vi "SELECCION_MODO_INGENIERIA.vi"(7 "EST_3":bool, 8 "EST_2":bool, 9 "EST_1":bool) -> (3 "MOV eSTADO":i32)   [LabVIEW 2019, in "Class 2.lvclass"]
uses:
  Class 2.lvclass
panel:
  out "ESTADO":i8
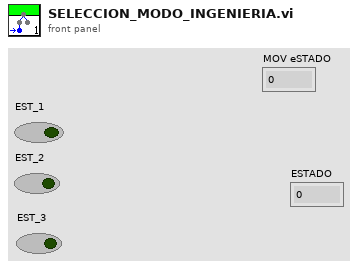
[diagram p1: front panel]
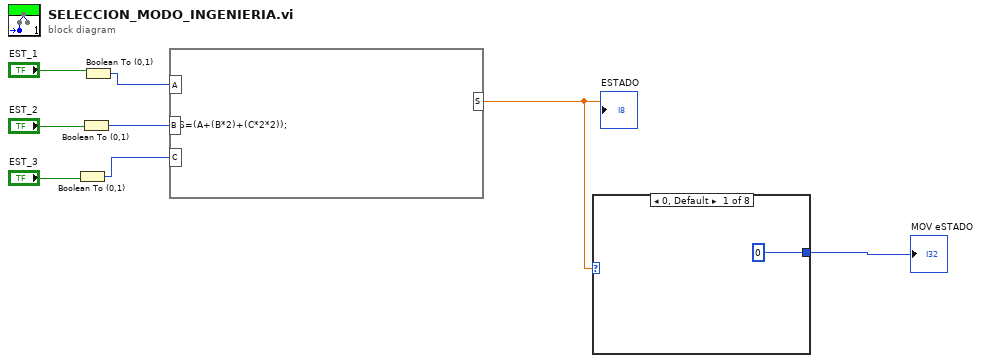
[diagram p0: block diagram]
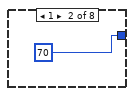
[diagram p2: hidden frame]
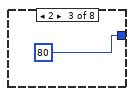
[diagram p3: hidden frame]
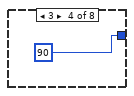
[diagram p4: hidden frame]
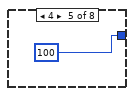
[diagram p5: hidden frame]
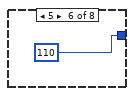
[diagram p6: hidden frame]
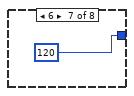
[diagram p7: hidden frame]
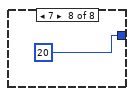
[diagram p8: hidden frame]
diagram:
  n1 = Boolean To (0,1)(Boolean="EST_3") -> (0, 1=w3:i16)
  n2 = Boolean To (0,1)(Boolean="EST_2") -> (0, 1=w4:i16)
  n3 = Boolean To (0,1)(Boolean="EST_1") -> (0, 1=w5:i16)
  n4 = formula code="S=(A+(B*2)+(C*2*2));"("A"=w5, "B"=w4, "C"=w3) -> ("S"=w2:dbl)
  "ESTADO" <- w2
  n5 = case shown="0, Default" w2 {
    tunnel: [0 70 80 90 100 110 120 20] -> w1
    frame 0, Default {
    }
    frame 1 {
    }
    frame 2 {
    }
    frame 3 {
    }
    frame 4 {
    }
    frame 5 {
    }
    frame 6 {
    }
    frame 7 {
    }
  }
  "MOV eSTADO" <- w1
